vi "digitalLevelToBool.vi"(11 "Digital Signal Level":T1) -> (3 "Bool?":bool)   [LabVIEW 2015]
uses:
  Typedefs/Digital Signal Level.ctl
  Typedefs/ILCBTTypedefs.lvlib
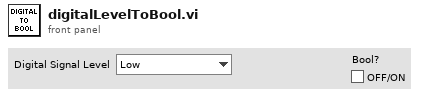
[diagram p1: front panel]
types:
  T1 = typedef "ILCBTTypedefs.lvlib/Digital Signal Level.ctl" = enum16{"Low", "High"}
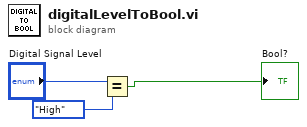
[diagram p0: block diagram]
diagram:
  n1 = Equal?(x="Digital Signal Level", y=Digital_Signal_Level."High") -> (x = y?=→"Bool?":bool)
